vi "Open Report.vi"(8 "error in":errorcluster, 11 "Report Viewer in":refnum<class "Report Viewer.lvclass">) -> (0 "error out":errorcluster, 3 "Report Viewer out":refnum<class "Report Viewer.lvclass">)   [LabVIEW 2023, in "Report Viewer.lvlib" / "Report Viewer.lvclass"]
uses:
  Library/Report Viewer.lvclass
  Library/Report Viewer.lvclass/Report Viewer.ctl
  Accessors/Write TDMS_Path.vi
  Accessors/Write tdms file ref.vi
  Private/Update File Name.vi
  Private/Tree/Insert File Content.vi
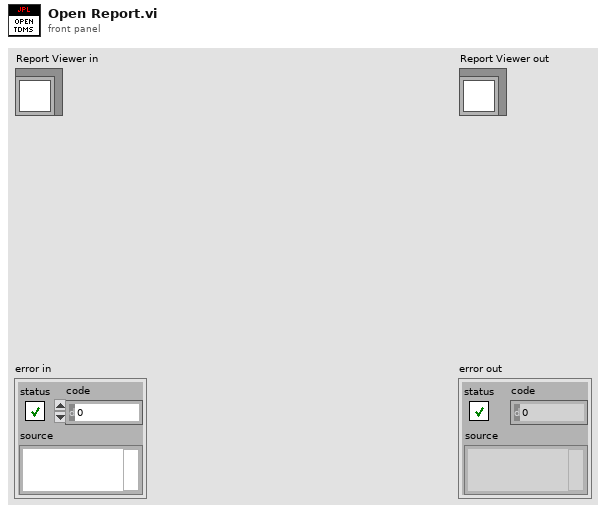
[diagram p1: front panel]
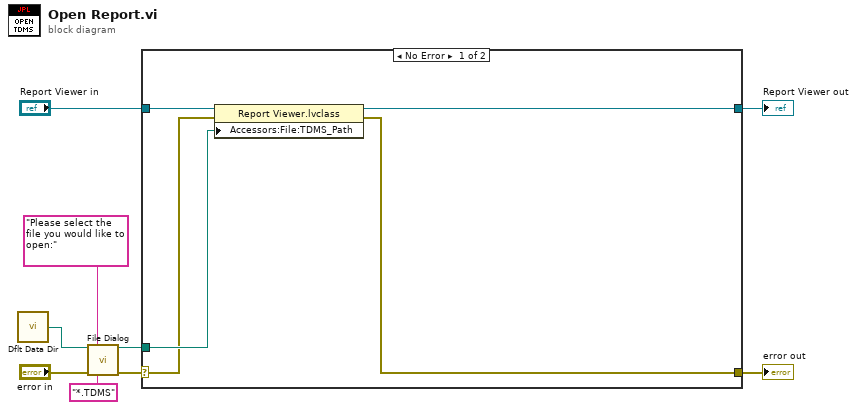
[diagram p0: block diagram]
diagram:
  n1 = call <vilib>:"Dflt Data Dir.vi"() -> ("App:Default Data Directory"=w6:path)
  n2 = call "File Dialog"("start path"=w6, "prompt"="Please select the file you would like to open:", "error in"="error in", "pattern (all files)"="*.TDMS") -> ("selected path"=w3:path, "error out"=w4:errorcluster)  [unwired: 8 in, 2 out]
  n3 = case shown="No Error" w4 {
    selector: w4 -> [w12 _]
    tunnel: [w11 _] -> w9
    tunnel: [w10 w15] -> w7
    tunnel: "Report Viewer in" -> [w14 w15]
    tunnel: w3 -> [w13 _]
    frame No Error {
      n4 = property class="Report Viewer.lvclass"(reference=w14, error in=w12, "Accessors:File:TDMS_Path"=w13) -> (reference out=w10:refnum<class "Report Viewer.lvclass">, error out=w11:errorcluster)
    }
    frame Error {
    }
  }
  "error out" <- w9
  "Report Viewer out" <- w7
